vi "_emi_create version id file.vi"(0 "vi Refnum in":refnum<vi>, 7 "Version Filename string":string, 11 "error in":errorcluster) -> (4 "vi Refnum out":refnum<vi>, 15 "error out":errorcluster)   [LabVIEW 2010]
doc: "Creates a *.ver file, in the same directory as the VI connected in the vi Refnum in.\n\nDoes not generate a new error, if eerro in, does noe execute"
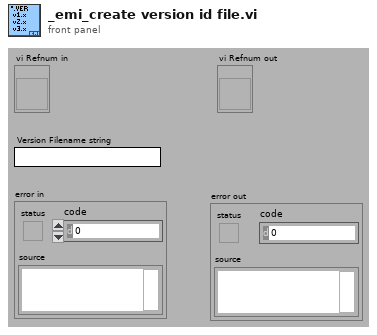
[diagram p1: front panel]
types:
  T1 = enum16{"open", "replace", "create", "open or create", "replace or create", "replace or create with confirmation"}
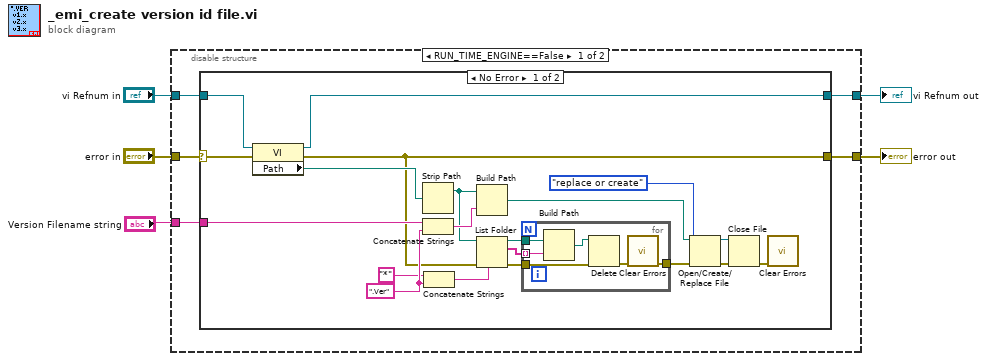
[diagram p0: block diagram]
diagram:
  n1 = disable-structure shown="RUN_TIME_ENGINE==False" {
    disable-tunnel: [w10 w40] -> w5
    disable-tunnel: "vi Refnum in" -> [w9 w40]
    disable-tunnel: "Version Filename string" -> [w8 _]
    disable-tunnel: [w7 w39] -> w2
    disable-tunnel: "error in" -> [w6 w39]
    frame condition #0 (active) {
      n2 = case shown="No Error" w6 {
        selector: w6 -> [w11 w37]
        tunnel: [w29 w38] -> w10
        tunnel: w9 -> [w28 w38]
        tunnel: w8 -> [w26 _]
        tunnel: [w12 w37] -> w7
        frame No Error {
          w24 = ".Ver" ("string")
          n3 = property class="VI"(reference=w28, error in=w11) -> (reference out=w29:refnum<vi>, error out=w12:errorcluster, "Path"=w30:path)
          n4 = Strip Path(path=w30) -> (stripped path=w21:path)  [unwired: 1 out]
          n5 = Concatenate Strings(w26, w24) -> (w25:string)
          n6 = Concatenate Strings("*" ("string"), w24) -> (w22:string)
          n7 = Build Path(base path=w21, name or relative path=w25) -> (appended path=w27:path)
          n8 = List Folder(path=w21, pattern=w22, error in=w12) -> (path out=w19:path, filenames=w18:string[], error out=w20:errorcluster)  [unwired: 1 in, 1 out]
          n9 = for {
            tunnel: w20 -> [w36]
            tunnel: w19 -> [w35]
            tunnel: w18 -> [w34] mode=indexing
            tunnel: [w31] -> w14
            n10 = Build Path(base path=w35, name or relative path=w34) -> (appended path=w32:path)
            n11 = Delete(path (use dialog)=w32, error in=w36) -> (error out=w33:errorcluster)  [unwired: 3 in, 2 out]
            n12 = call <vilib>:"Clear Errors.vi"("error in (no error)"=w33) -> ("error out"=w31:errorcluster)  [unwired: 6 in]
          }
          n13 = Open/Create/Replace File(file path (use dialog)=w27, error in=w14, operation (0:open)=T1."replace or create") -> (refnum out=w17:refnum<file>, error out=w15:errorcluster)  [unwired: 3 in, 1 out]
          n14 = Close File(refnum=w17, error in=w15) -> (error out=w13:errorcluster)  [unwired: 1 out]
          n15 = call <vilib>:"Clear Errors.vi"("error in (no error)"=w13) -> ()  [unwired: 6 in, 1 out]
        }
        frame Error {
        }
      }
    }
    frame condition #1 {
    }
  }
  "error out" <- w2
  "vi Refnum out" <- w5
